vi "Autonomous Independent.vi"() -> ()   [LabVIEW 2013]
doc: "This VI is called when autonomous begins, and will automatically be terminated when autonomous ends. You can carry out timed or sensor driven robot movement independently without needing to return to the caller."
uses:
  Systems/DriveMotors/DriveMotors.lvclass
  Systems/GrabberWheels/GrabberWheels.lvclass
  Systems/GrabberArms/GrabberArms.lvclass
  Commands/Command/Command.lvclass
  Systems/Catapult/Catapult.lvclass
  Commands/CT-De-energize-Command/CT-De-energize-Cmd.lvclass
  Systems/Blocker/Blocker.lvclass
  Commands/DM-DriveForwardDistance/DM-DriveForwardDistance.lvclass
  Robot Global Data.vi
  Commands/GA-Extend-Command/GA-Extend-Cmd.lvclass
  Commands/BL-Extend-Command/BL-Extend-Cmd.lvclass
  Commands/GW-SpitOut-Command/GW-SpitOut-Cmd.lvclass
  Commands/GW-Stop-Command/GW-Stop-Cmd.lvclass
panel:
  in  "Time to Settle(ms)":u32=500
  in  "Time to Spit Out":u32
  out "AutoMode: Drive Forward and Shoot":bool
  in  "Use PID":bool
  out "Right Power":dbl
  in  "Trim":dbl(knob) step=0.001 scale=0.0..0.25
  in  "Test Wait":u32=25
  in  "DrivePower":dbl=0.6 format="%#_13g"
  # "Be sure to right-click and choose Data Operations>>Make Current Value default if you want to save the array values with the VI"
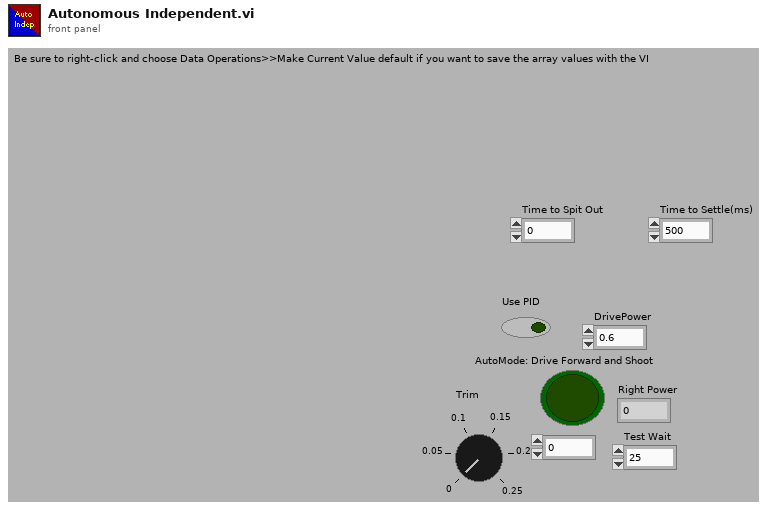
[diagram p1: front panel]
types:
  T1 = typedef "Semaphore RefNum" = refnum<k1>
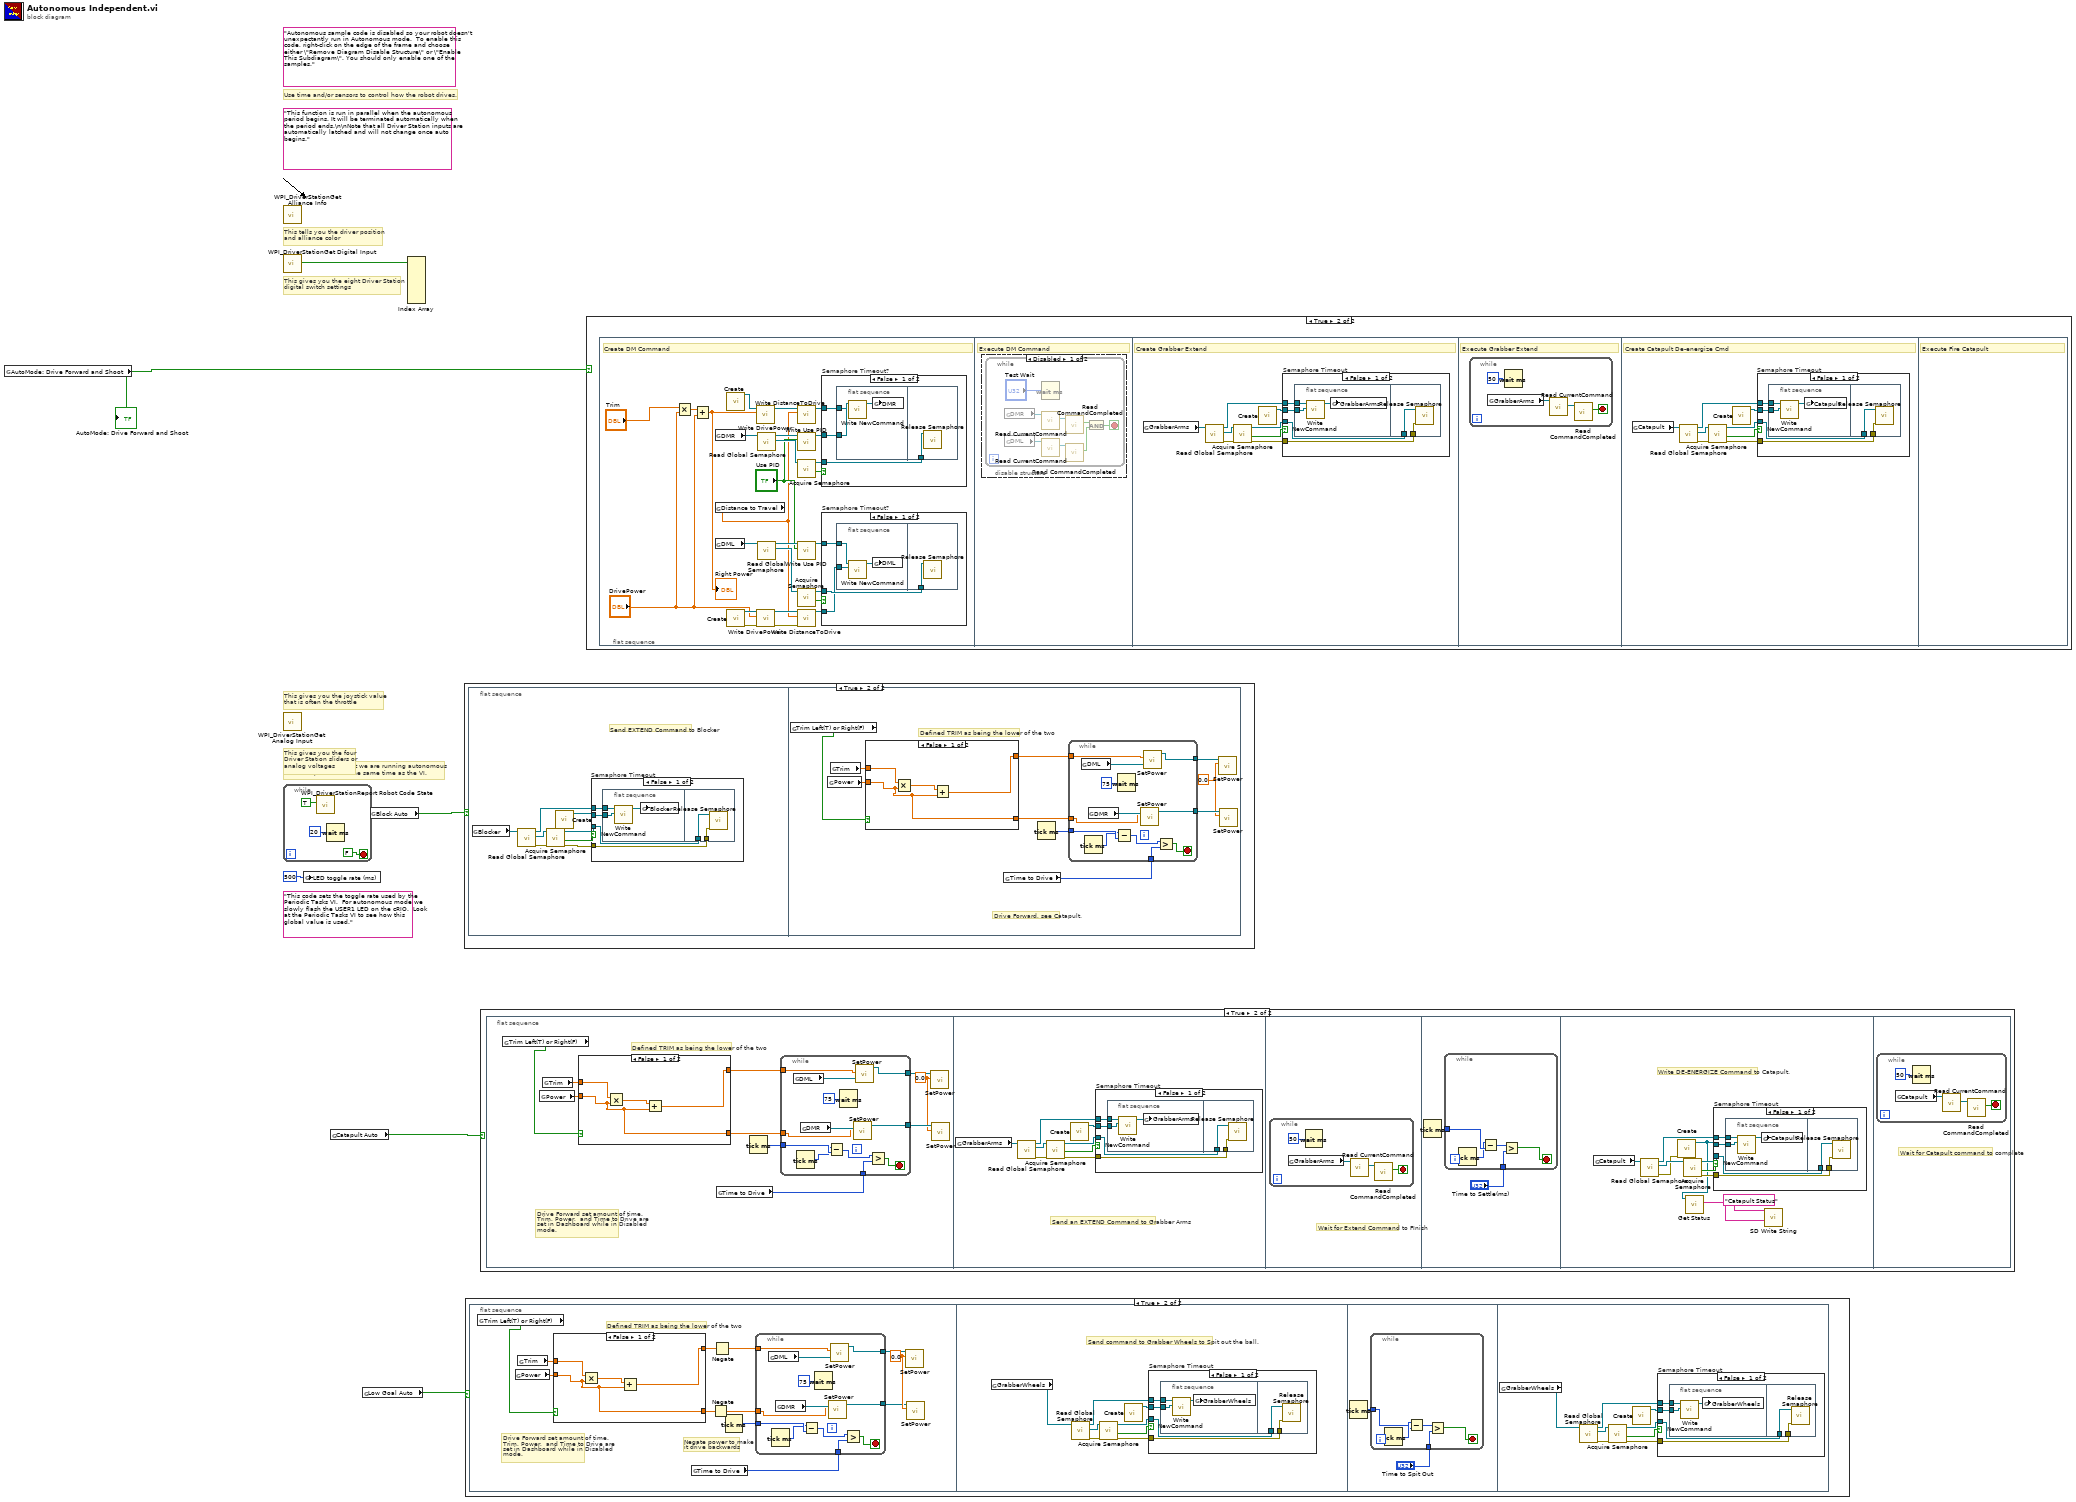
[diagram p0: block diagram]
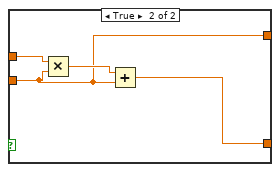
[diagram p3: hidden frame]
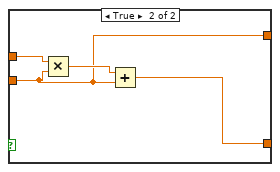
[diagram p7: hidden frame]
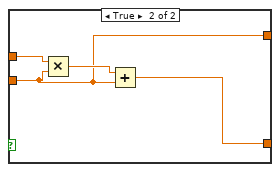
[diagram p12: hidden frame]
diagram:
  (unwired) "This code sets the toggle rate used by the Periodic Tasks VI.  For autonomous mode we slowly flash the USER1 LED on the cRIO.  Look at the Periodic Tasks VI to see how this global value is used."
  (unwired) "Autonomous sample code is disabled so your robot doesn't unexpectantly run in Autonomous mode.  To enable this code, right-click on the edge of the frame and choose either \"Remove Diagram Disable Structure\" or \"Enable This Subdiagram\". You should only enable one of the samples."
  (unwired) "This function is run in parallel when the autonomous period begins. It will be terminated automatically when the period ends.\n\nNote that all Driver Station inputs are automatically latched and will not change once auto begins."
  # "Every 20ms, report that we are running autonomous\ncode. Loop will abort the same time as the VI."
  # "This gives you the joystick value\nthat is often the throttle"
  # "Use time and/or sensors to control how the robot drives."
  # "This tells you the driver position\nand alliance color"
  # "This gives you the eight Driver Station\ndigital switch settings"
  # "This gives you the four\nDriver Station sliders or\nanalog voltages"
  n1 = global read "Robot Global Data.vi" "AutoMode: Drive Forward and Shoot"() -> (w4:bool)
  "AutoMode: Drive Forward and Shoot" <- w4
  n2 = call <vilib>:"WPI_DriverStationGet Alliance Info.vi"() -> ()  [unwired: 12 out]
  n3 = call <vilib>:"WPI_DriverStationGet Digital Input.vi"() -> ("Driver Station Digital Input (1-8)"=w6:bool[])  [unwired: 11 out]
  n4 = call <vilib>:"WPI_DriverStationGet Analog Input.vi"() -> ()  [unwired: 12 out]
  n5 = while {
    stop <- FALSE stop-if-true
    n6 = call <vilib>:"WPI_DriverStationReport Robot Code State.vi"("Autonomous"=TRUE) -> ()  [unwired: 10 in, 1 out]
    n7 = Wait (ms)(milliseconds to wait=u32 20) -> ()  [unwired: 1 out]
  }
  n8 = global write "Robot Global Data.vi" "LED toggle rate (ms)"(u32 500 ("LED ms toggle rate")) -> ()
  n9 = global read "Robot Global Data.vi" "Catapult Auto"() -> (w2:bool)
  n10 = global read "Robot Global Data.vi" "Low Goal Auto"() -> (w1:bool)
  n11 = global read "Robot Global Data.vi" "Block Auto"() -> (w3:bool)
  n12 = Index Array(array=w6) -> ()  [unwired: 8 in, 8 out]
  n13 = case shown="True" w3 {
    frame False {
    }
    frame True {
      n14 = flat-sequence {
        frame #0 {
          # "Send EXTEND Command to Blocker"
          n15 = global read "Robot Global Data.vi" "Blocker"() -> (w17:refnum<class "Blocker.lvclass">)
          n16 = call-dynamic "Read Global Semaphore.vi"("System in"=w17) -> ("error out"=w14:errorcluster, "semaphore"=w15:T1, "System out"=w16:refnum<class "Blocker.lvclass">)  [unwired: 8 in]
          n17 = call <vilib>:"Acquire Semaphore.vi"("error in (no error)"=w14, "semaphore"=w15) -> ("error out"=w12:errorcluster, "timed out"=w11:bool, "semaphore out"=w13:T1)  [unwired: 3 in]
          n18 = call "Create.vi"() -> ("BL-Extend-Cmd out"=w10:refnum<class "BL-Extend-Cmd.lvclass">)  [unwired: 10 in, 1 out]
          n19 = case "Semaphore Timeout" shown="False" w11 {
            tunnel: w16 -> [w21 _]
            tunnel: w13 -> [w20 _]
            tunnel: w12 -> [w19 _]
            tunnel: w10 -> [w18 _]
            frame False {
              n20 = flat-sequence {
                tunnel: w21 -> [w23]
                tunnel: w18 -> [w22]
                tunnel: w20 -> [w26]
                tunnel: w19 -> [w25]
                frame #0 {
                  n21 = call-dynamic "Write NewCommand.vi"("Command.lvclass"=w22, "System in"=w23) -> ("System out"=w24:refnum<class "Blocker.lvclass">)  [unwired: 8 in, 1 out]
                  n22 = global write "Robot Global Data.vi" "Blocker"(w24) -> ()
                }
                frame #1 {
                  n23 = call <vilib>:"Release Semaphore.vi"("error in (no error)"=w25, "semaphore"=w26) -> ()  [unwired: 4 in, 2 out]
                }
              }
            }
            frame True {
            }
          }
        }
        frame #1 {
          w33 = 0.0 ("MotorPower Terminal")
          # "Drive Forward, see Catapult."
          # "Defined TRIM as being the lower of the two"
          n24 = global read "Robot Global Data.vi" "Trim Left(T) or Right(F)"() -> (w32:bool)
          n25 = global read "Robot Global Data.vi" "Power"() -> (w30:dbl)
          n26 = global read "Robot Global Data.vi" "Trim"() -> (w31:dbl)
          n27 = case shown="False" w32 {
            tunnel: w31 -> [w39 w44]
            tunnel: w30 -> [w37 w41]
            tunnel: [w37 w42] -> w29
            tunnel: [w38 w41] -> w28
            frame False {
              n28 = Multiply(x=w39, y=w37) -> (x*y=w40:dbl)
              n29 = Add(x=w40, y=w37) -> (x+y=w38:dbl)
            }
            frame True {
              n30 = Multiply(x=w44, y=w41) -> (x*y=w43:dbl)
              n31 = Add(x=w43, y=w41) -> (x+y=w42:dbl)
            }
          }
          n32 = global read "Robot Global Data.vi" "Time to Drive"() -> (w27:u32)
          n33 = Tick Count (ms)() -> (millisecond timer value=w36:u32)
          n34 = while {
            tunnel: w36 -> [w54]
            tunnel: [w51] -> w35
            tunnel: [w50] -> w34
            tunnel: w29 -> [w48]
            tunnel: w28 -> [w47]
            tunnel: w27 -> [w46]
            stop <- w49 stop-if-true
            n35 = global read "Robot Global Data.vi" "DML"() -> (w55:refnum<class "DriveMotors.lvclass">)
            n36 = Tick Count (ms)() -> (millisecond timer value=w53:u32)
            n37 = global read "Robot Global Data.vi" "DMR"() -> (w56:refnum<class "DriveMotors.lvclass">)
            n38 = Subtract(x=w53, y=w54) -> (x-y=w52:u32)
            n39 = Wait (ms)(milliseconds to wait=u32 75) -> ()  [unwired: 1 out]
            n40 = call-dynamic "SetPower.vi"("MotorPower Terminal"=w48, "DriveMotors in"=w56) -> ("DriveMotors out"=w51:refnum<class "DriveMotors.lvclass">)  [unwired: 8 in, 1 out]
            n41 = call-dynamic "SetPower.vi"("MotorPower Terminal"=w47, "DriveMotors in"=w55) -> ("DriveMotors out"=w50:refnum<class "DriveMotors.lvclass">)  [unwired: 8 in, 1 out]
            n42 = Greater?(x=w52, y=w46) -> (0:w49:bool)
          }
          n43 = call-dynamic "SetPower.vi"("MotorPower Terminal"=w33, "DriveMotors in"=w34) -> ()  [unwired: 8 in, 2 out]
          n44 = call-dynamic "SetPower.vi"("MotorPower Terminal"=w33, "DriveMotors in"=w35) -> ()  [unwired: 8 in, 2 out]
        }
      }
    }
  }
  n45 = case shown="True" w1 {
    frame False {
    }
    frame True {
      n46 = flat-sequence {
        frame #0 {
          w62 = 0.0 ("MotorPower Terminal")
          # "Negate power to make \nit drive backwards"
          # "Drive Forward set amount of time.\nTrim, Power,  and Time to Drive are \nset in Dashboard while in Disabled \nmode."
          # "Defined TRIM as being the lower of the two"
          n47 = global read "Robot Global Data.vi" "Trim Left(T) or Right(F)"() -> (w63:bool)
          n48 = global read "Robot Global Data.vi" "Power"() -> (w65:dbl)
          n49 = global read "Robot Global Data.vi" "Trim"() -> (w64:dbl)
          n50 = case shown="False" w63 {
            tunnel: w64 -> [w71 w76]
            tunnel: w65 -> [w69 w73]
            tunnel: [w69 w74] -> w66
            tunnel: [w70 w73] -> w67
            frame False {
              n51 = Multiply(x=w71, y=w69) -> (x*y=w72:dbl)
              n52 = Add(x=w72, y=w69) -> (x+y=w70:dbl)
            }
            frame True {
              n53 = Multiply(x=w76, y=w73) -> (x*y=w75:dbl)
              n54 = Add(x=w75, y=w73) -> (x+y=w74:dbl)
            }
          }
          n55 = global read "Robot Global Data.vi" "Time to Drive"() -> (w68:u32)
          n56 = Negate(x=w66) -> (-x=w57:dbl)
          n57 = Negate(x=w67) -> (-x=w58:dbl)
          n58 = Tick Count (ms)() -> (millisecond timer value=w59:u32)
          n59 = while {
            tunnel: w59 -> [w86]
            tunnel: [w83] -> w60
            tunnel: [w82] -> w61
            tunnel: w57 -> [w80]
            tunnel: w58 -> [w79]
            tunnel: w68 -> [w78]
            stop <- w81 stop-if-true
            n60 = global read "Robot Global Data.vi" "DML"() -> (w87:refnum<class "DriveMotors.lvclass">)
            n61 = Tick Count (ms)() -> (millisecond timer value=w85:u32)
            n62 = global read "Robot Global Data.vi" "DMR"() -> (w88:refnum<class "DriveMotors.lvclass">)
            n63 = Subtract(x=w85, y=w86) -> (x-y=w84:u32)
            n64 = Wait (ms)(milliseconds to wait=u32 75) -> ()  [unwired: 1 out]
            n65 = call-dynamic "SetPower.vi"("MotorPower Terminal"=w80, "DriveMotors in"=w88) -> ("DriveMotors out"=w83:refnum<class "DriveMotors.lvclass">)  [unwired: 8 in, 1 out]
            n66 = call-dynamic "SetPower.vi"("MotorPower Terminal"=w79, "DriveMotors in"=w87) -> ("DriveMotors out"=w82:refnum<class "DriveMotors.lvclass">)  [unwired: 8 in, 1 out]
            n67 = Greater?(x=w84, y=w78) -> (0:w81:bool)
          }
          n68 = call-dynamic "SetPower.vi"("MotorPower Terminal"=w62, "DriveMotors in"=w61) -> ()  [unwired: 8 in, 2 out]
          n69 = call-dynamic "SetPower.vi"("MotorPower Terminal"=w62, "DriveMotors in"=w60) -> ()  [unwired: 8 in, 2 out]
        }
        frame #1 {
          # "Send command to Grabber Wheels to Spit out the ball."
          n70 = global read "Robot Global Data.vi" "GrabberWheels"() -> (w89:refnum<class "GrabberWheels.lvclass">)
          n71 = call-dynamic "Read Global Semaphore.vi"("System in"=w89) -> ("error out"=w92:errorcluster, "semaphore"=w91:T1, "System out"=w90:refnum<class "GrabberWheels.lvclass">)  [unwired: 8 in]
          n72 = call <vilib>:"Acquire Semaphore.vi"("error in (no error)"=w92, "semaphore"=w91) -> ("error out"=w95:errorcluster, "timed out"=w93:bool, "semaphore out"=w94:T1)  [unwired: 3 in]
          n73 = call "Create.vi"() -> ("GW-SpitOut-Cmd out"=w96:refnum<class "GW-SpitOut-Cmd.lvclass">)  [unwired: 10 in, 1 out]
          n74 = case "Semaphore Timeout" shown="False" w93 {
            tunnel: w90 -> [w100 _]
            tunnel: w94 -> [w99 _]
            tunnel: w95 -> [w98 _]
            tunnel: w96 -> [w97 _]
            frame False {
              n75 = flat-sequence {
                tunnel: w100 -> [w102]
                tunnel: w97 -> [w101]
                tunnel: w99 -> [w105]
                tunnel: w98 -> [w104]
                frame #0 {
                  n76 = call-dynamic "Write NewCommand.vi"("Command.lvclass"=w101, "System in"=w102) -> ("System out"=w103:refnum<class "GrabberWheels.lvclass">)  [unwired: 8 in, 1 out]
                  n77 = global write "Robot Global Data.vi" "GrabberWheels"(w103) -> ()
                }
                frame #1 {
                  n78 = call <vilib>:"Release Semaphore.vi"("error in (no error)"=w104, "semaphore"=w105) -> ()  [unwired: 4 in, 2 out]
                }
              }
            }
            frame True {
            }
          }
        }
        frame #2 {
          n79 = Tick Count (ms)() -> (millisecond timer value=w107:u32)
          n80 = while {
            tunnel: w107 -> [w108]
            tunnel: "Time to Spit Out" -> [w110]
            stop <- w111 stop-if-true
            n81 = Tick Count (ms)() -> (millisecond timer value=w109:u32)
            n82 = Subtract(x=w109, y=w108) -> (x-y=w112:u32)
            n83 = Greater?(x=w112, y=w110) -> (0:w111:bool)
          }
        }
        frame #3 {
          n84 = global read "Robot Global Data.vi" "GrabberWheels"() -> (w113:refnum<class "GrabberWheels.lvclass">)
          n85 = call-dynamic "Read Global Semaphore.vi"("System in"=w113) -> ("error out"=w116:errorcluster, "semaphore"=w115:T1, "System out"=w114:refnum<class "GrabberWheels.lvclass">)  [unwired: 8 in]
          n86 = call <vilib>:"Acquire Semaphore.vi"("error in (no error)"=w116, "semaphore"=w115) -> ("error out"=w119:errorcluster, "timed out"=w117:bool, "semaphore out"=w118:T1)  [unwired: 3 in]
          n87 = call "Create.vi"() -> ("GW-Stop-Cmd out"=w120:refnum<class "GW-Stop-Cmd.lvclass">)  [unwired: 10 in, 1 out]
          n88 = case "Semaphore Timeout" shown="False" w117 {
            tunnel: w114 -> [w124 _]
            tunnel: w118 -> [w123 _]
            tunnel: w119 -> [w122 _]
            tunnel: w120 -> [w121 _]
            frame False {
              n89 = flat-sequence {
                tunnel: w124 -> [w126]
                tunnel: w121 -> [w125]
                tunnel: w123 -> [w129]
                tunnel: w122 -> [w128]
                frame #0 {
                  n90 = call-dynamic "Write NewCommand.vi"("Command.lvclass"=w125, "System in"=w126) -> ("System out"=w127:refnum<class "GrabberWheels.lvclass">)  [unwired: 8 in, 1 out]
                  n91 = global write "Robot Global Data.vi" "GrabberWheels"(w127) -> ()
                }
                frame #1 {
                  n92 = call <vilib>:"Release Semaphore.vi"("error in (no error)"=w128, "semaphore"=w129) -> ()  [unwired: 4 in, 2 out]
                }
              }
            }
            frame True {
            }
          }
        }
      }
    }
  }
  n93 = case shown="True" w2 {
    frame False {
    }
    frame True {
      n94 = flat-sequence {
        frame #0 {
          w136 = 0.0 ("MotorPower Terminal")
          # "Drive Forward set amount of time.\nTrim, Power,  and Time to Drive are \nset in Dashboard while in Disabled \nmode."
          # "Defined TRIM as being the lower of the two"
          n95 = global read "Robot Global Data.vi" "Trim Left(T) or Right(F)"() -> (w135:bool)
          n96 = global read "Robot Global Data.vi" "Power"() -> (w133:dbl)
          n97 = global read "Robot Global Data.vi" "Trim"() -> (w134:dbl)
          n98 = case shown="False" w135 {
            tunnel: w134 -> [w142 w147]
            tunnel: w133 -> [w140 w144]
            tunnel: [w140 w145] -> w132
            tunnel: [w141 w144] -> w131
            frame False {
              n99 = Multiply(x=w142, y=w140) -> (x*y=w143:dbl)
              n100 = Add(x=w143, y=w140) -> (x+y=w141:dbl)
            }
            frame True {
              n101 = Multiply(x=w147, y=w144) -> (x*y=w146:dbl)
              n102 = Add(x=w146, y=w144) -> (x+y=w145:dbl)
            }
          }
          n103 = global read "Robot Global Data.vi" "Time to Drive"() -> (w130:u32)
          n104 = Tick Count (ms)() -> (millisecond timer value=w139:u32)
          n105 = while {
            tunnel: w139 -> [w157]
            tunnel: [w154] -> w138
            tunnel: [w153] -> w137
            tunnel: w132 -> [w151]
            tunnel: w131 -> [w150]
            tunnel: w130 -> [w149]
            stop <- w152 stop-if-true
            n106 = global read "Robot Global Data.vi" "DML"() -> (w158:refnum<class "DriveMotors.lvclass">)
            n107 = Tick Count (ms)() -> (millisecond timer value=w156:u32)
            n108 = global read "Robot Global Data.vi" "DMR"() -> (w159:refnum<class "DriveMotors.lvclass">)
            n109 = Subtract(x=w156, y=w157) -> (x-y=w155:u32)
            n110 = Wait (ms)(milliseconds to wait=u32 75) -> ()  [unwired: 1 out]
            n111 = call-dynamic "SetPower.vi"("MotorPower Terminal"=w151, "DriveMotors in"=w159) -> ("DriveMotors out"=w154:refnum<class "DriveMotors.lvclass">)  [unwired: 8 in, 1 out]
            n112 = call-dynamic "SetPower.vi"("MotorPower Terminal"=w150, "DriveMotors in"=w158) -> ("DriveMotors out"=w153:refnum<class "DriveMotors.lvclass">)  [unwired: 8 in, 1 out]
            n113 = Greater?(x=w155, y=w149) -> (0:w152:bool)
          }
          n114 = call-dynamic "SetPower.vi"("MotorPower Terminal"=w136, "DriveMotors in"=w137) -> ()  [unwired: 8 in, 2 out]
          n115 = call-dynamic "SetPower.vi"("MotorPower Terminal"=w136, "DriveMotors in"=w138) -> ()  [unwired: 8 in, 2 out]
        }
        frame #1 {
          # "Send an EXTEND Command to Grabber Arms"
          n116 = global read "Robot Global Data.vi" "GrabberArms"() -> (w167:refnum<class "GrabberArms.lvclass">)
          n117 = call-dynamic "Read Global Semaphore.vi"("System in"=w167) -> ("error out"=w164:errorcluster, "semaphore"=w165:T1, "System out"=w166:refnum<class "GrabberArms.lvclass">)  [unwired: 8 in]
          n118 = call <vilib>:"Acquire Semaphore.vi"("error in (no error)"=w164, "semaphore"=w165) -> ("error out"=w161:errorcluster, "timed out"=w163:bool, "semaphore out"=w162:T1)  [unwired: 3 in]
          n119 = call "Create.vi"() -> ("GA-Extend-Cmd out"=w160:refnum<class "GA-Extend-Cmd.lvclass">)  [unwired: 10 in, 1 out]
          n120 = case "Semaphore Timeout" shown="False" w163 {
            tunnel: w166 -> [w171 _]
            tunnel: w162 -> [w170 _]
            tunnel: w161 -> [w169 _]
            tunnel: w160 -> [w168 _]
            frame False {
              n121 = flat-sequence {
                tunnel: w171 -> [w173]
                tunnel: w168 -> [w172]
                tunnel: w170 -> [w176]
                tunnel: w169 -> [w175]
                frame #0 {
                  n122 = call-dynamic "Write NewCommand.vi"("Command.lvclass"=w172, "System in"=w173) -> ("System out"=w174:refnum<class "GrabberArms.lvclass">)  [unwired: 8 in, 1 out]
                  n123 = global write "Robot Global Data.vi" "GrabberArms"(w174) -> ()
                }
                frame #1 {
                  n124 = call <vilib>:"Release Semaphore.vi"("error in (no error)"=w175, "semaphore"=w176) -> ()  [unwired: 4 in, 2 out]
                }
              }
            }
            frame True {
            }
          }
        }
        frame #2 {
          # "Wait for Extend Command to FInish"
          n125 = while {
            stop <- w177 stop-if-true
            n126 = global read "Robot Global Data.vi" "GrabberArms"() -> (w178:refnum<class "GrabberArms.lvclass">)
            n127 = Wait (ms)(milliseconds to wait=u32 50) -> ()  [unwired: 1 out]
            n128 = call-dynamic "Read CurrentCommand.vi"("System in"=w178) -> ("Command.lvclass"=w179:refnum<class "Command.lvclass">)  [unwired: 8 in, 2 out]
            n129 = call-dynamic "Read CommandCompleted.vi"("Command in"=w179) -> ("CommandCompleted"=w177:bool)  [unwired: 8 in, 2 out]
          }
        }
        frame #3 {
          n130 = Tick Count (ms)() -> (millisecond timer value=w182:u32)
          n131 = while {
            tunnel: w182 -> [w184]
            tunnel: "Time to Settle(ms)" -> [w185]
            stop <- w186 stop-if-true
            n132 = Tick Count (ms)() -> (millisecond timer value=w183:u32)
            n133 = Subtract(x=w183, y=w184) -> (x-y=w187:u32)
            n134 = Greater?(x=w187, y=w185) -> (0:w186:bool)
          }
        }
        frame #4 {
          # "Write DE-ENERGIZE Command to Catapult."
          n135 = global read "Robot Global Data.vi" "Catapult"() -> (w198:refnum<class "Catapult.lvclass">)
          n136 = call-dynamic "Read Global Semaphore.vi"("System in"=w198) -> ("error out"=w189:errorcluster, "semaphore"=w196:T1, "System out"=w197:refnum<class "Catapult.lvclass">)  [unwired: 8 in]
          n137 = call "Create.vi"("error in (no error)"=w189) -> ("error out"=w188:errorcluster, "CT-De-energize-Cmd.lvclass"=w192:refnum<class "CT-De-energize-Cmd.lvclass">)  [unwired: 9 in]
          n138 = call <vilib>:"Acquire Semaphore.vi"("error in (no error)"=w188, "semaphore"=w196) -> ("error out"=w194:errorcluster, "timed out"=w193:bool, "semaphore out"=w195:T1)  [unwired: 3 in]
          n139 = call-dynamic "Get Status.vi"("Command in"=w192) -> ("Status"=w191:string)  [unwired: 8 in, 2 out]
          n140 = case "Semaphore Timeout" shown="False" w193 {
            tunnel: w197 -> [w202 _]
            tunnel: w195 -> [w201 _]
            tunnel: w194 -> [w200 _]
            tunnel: w192 -> [w199 _]
            frame False {
              n141 = flat-sequence {
                tunnel: w202 -> [w204]
                tunnel: w199 -> [w203]
                tunnel: w201 -> [w207]
                tunnel: w200 -> [w206]
                frame #0 {
                  n142 = call-dynamic "Write NewCommand.vi"("Command.lvclass"=w203, "System in"=w204) -> ("System out"=w205:refnum<class "Catapult.lvclass">)  [unwired: 8 in, 1 out]
                  n143 = global write "Robot Global Data.vi" "Catapult"(w205) -> ()
                }
                frame #1 {
                  n144 = call <vilib>:"Release Semaphore.vi"("error in (no error)"=w206, "semaphore"=w207) -> ()  [unwired: 4 in, 2 out]
                }
              }
            }
            frame True {
            }
          }
          n145 = call <vilib>:"SD Write String.vi"("String"=w191, "Name"="Catapult Status") -> ()  [unwired: 8 in, 2 out]
        }
        frame #5 {
          # "Wait for Catapult command to complete"
          n146 = while {
            stop <- w208 stop-if-true
            n147 = global read "Robot Global Data.vi" "Catapult"() -> (w209:refnum<class "Catapult.lvclass">)
            n148 = Wait (ms)(milliseconds to wait=u32 50) -> ()  [unwired: 1 out]
            n149 = call-dynamic "Read CurrentCommand.vi"("System in"=w209) -> ("Command.lvclass"=w210:refnum<class "Command.lvclass">)  [unwired: 8 in, 2 out]
            n150 = call-dynamic "Read CommandCompleted.vi"("Command in"=w210) -> ("CommandCompleted"=w208:bool)  [unwired: 8 in, 2 out]
          }
        }
      }
    }
  }
  n151 = case shown="True" w4 {
    frame False {
    }
    frame True {
      n152 = flat-sequence {
        frame #0 {
          # "Create DM Command"
          n153 = Multiply(x="Trim", y="DrivePower") -> (x*y=w219:dbl)
          n154 = Add(x=w219, y="DrivePower") -> (x+y=w218:dbl)
          "Right Power" <- w218
          n155 = global read "Robot Global Data.vi" "DMR"() -> (w235:refnum<class "DriveMotors.lvclass">)
          n156 = global read "Robot Global Data.vi" "Distance to Travel"() -> (w212:dbl)
          n157 = global read "Robot Global Data.vi" "DML"() -> (w229:refnum<class "DriveMotors.lvclass">)
          n158 = call "Create.vi"() -> ("DM-DriveForwardDistance.lvclass"=w224:refnum<class "DM-DriveForwardDistance.lvclass">)  [unwired: 10 in, 1 out]
          n159 = call "Create.vi"() -> ("error out"=w231:errorcluster, "DM-DriveForwardDistance.lvclass"=w237:refnum<class "DM-DriveForwardDistance.lvclass">)  [unwired: 10 in]
          n160 = call-dynamic "Write DrivePower.vi"("DrivePower"=w218, "DM-DriveForwardDistance in"=w224) -> ("DM-DriveForwardDistance out"=w223:refnum<class "DM-DriveForwardDistance.lvclass">)  [unwired: 8 in, 1 out]
          n161 = call-dynamic "Write DrivePower.vi"("error in (no error)"=w231, "DrivePower"="DrivePower", "DM-DriveForwardDistance in"=w237) -> ("error out"=w230:errorcluster, "DM-DriveForwardDistance out"=w236:refnum<class "DM-DriveForwardDistance.lvclass">)  [unwired: 7 in]
          n162 = call-dynamic "Read Global Semaphore.vi"("System in"=w235) -> ("semaphore"=w234:T1, "System out"=w217:refnum<class "DriveMotors.lvclass">)  [unwired: 8 in, 1 out]
          n163 = call-dynamic "Read Global Semaphore.vi"("System in"=w229) -> ("semaphore"=w228:T1, "System out"=w215:refnum<class "DriveMotors.lvclass">)  [unwired: 8 in, 1 out]
          n164 = call-dynamic "Write DistanceToDrive.vi"("DistanceToDrive"=w212, "DM-DriveForwardDistance in"=w223) -> ("DM-DriveForwardDistance out"=w222:refnum<class "DM-DriveForwardDistance.lvclass">)  [unwired: 8 in, 1 out]
          n165 = call-dynamic "Write Use PID.vi"("Use PID"="Use PID", "DriveMotors in"=w217) -> ("DriveMotors out"=w216:refnum<class "DriveMotors.lvclass">)  [unwired: 8 in, 1 out]
          n166 = call <vilib>:"Acquire Semaphore.vi"("semaphore"=w234) -> ("timed out"=w233:bool, "semaphore out"=w232:T1)  [unwired: 4 in, 1 out]
          n167 = call-dynamic "Write Use PID.vi"("Use PID"="Use PID", "DriveMotors in"=w215) -> ("DriveMotors out"=w214:refnum<class "DriveMotors.lvclass">)  [unwired: 8 in, 1 out]
          n168 = call <vilib>:"Acquire Semaphore.vi"("semaphore"=w228) -> ("timed out"=w226:bool, "semaphore out"=w227:T1)  [unwired: 4 in, 1 out]
          n169 = call-dynamic "Write DistanceToDrive.vi"("error in (no error)"=w230, "DistanceToDrive"=w212, "DM-DriveForwardDistance in"=w236) -> ("DM-DriveForwardDistance out"=w225:refnum<class "DM-DriveForwardDistance.lvclass">)  [unwired: 7 in, 1 out]
          n170 = case "Semaphore Timeout?" shown="False" w233 {
            tunnel: w216 -> [w247 _]
            tunnel: w222 -> [w246 _]
            tunnel: w232 -> [w245 _]
            frame False {
              n171 = flat-sequence {
                tunnel: w247 -> [w250]
                tunnel: w246 -> [w249]
                tunnel: w245 -> [w251]
                frame #0 {
                  n172 = call-dynamic "Write NewCommand.vi"("Command.lvclass"=w249, "System in"=w250) -> ("System out"=w248:refnum<class "DriveMotors.lvclass">)  [unwired: 8 in, 1 out]
                  n173 = global write "Robot Global Data.vi" "DMR"(w248) -> ()
                }
                frame #1 {
                  n174 = call <vilib>:"Release Semaphore.vi"("semaphore"=w251) -> ()  [unwired: 5 in, 2 out]
                }
              }
            }
            frame True {
            }
          }
          n175 = case "Semaphore Timeout?" shown="False" w226 {
            tunnel: w214 -> [w240 _]
            tunnel: w227 -> [w239 _]
            tunnel: w225 -> [w238 _]
            frame False {
              n176 = flat-sequence {
                tunnel: w240 -> [w243]
                tunnel: w238 -> [w242]
                tunnel: w239 -> [w244]
                frame #0 {
                  n177 = call-dynamic "Write NewCommand.vi"("Command.lvclass"=w242, "System in"=w243) -> ("System out"=w241:refnum<class "DriveMotors.lvclass">)  [unwired: 8 in, 1 out]
                  n178 = global write "Robot Global Data.vi" "DML"(w241) -> ()
                }
                frame #1 {
                  n179 = call <vilib>:"Release Semaphore.vi"("semaphore"=w244) -> ()  [unwired: 5 in, 2 out]
                }
              }
            }
            frame True {
            }
          }
        }
        frame #1 {
          # "Execute DM Command"
          n180 = disable-structure shown="Disabled" {
            frame Disabled {
              n181 = while {
                stop <- w253 stop-if-true
                n182 = global read "Robot Global Data.vi" "DMR"() -> (w256:refnum<class "DriveMotors.lvclass">)
                n183 = global read "Robot Global Data.vi" "DML"() -> (w255:refnum<class "DriveMotors.lvclass">)
                n184 = Wait (ms)(milliseconds to wait="Test Wait") -> ()  [unwired: 1 out]
                n185 = call-dynamic "Read CurrentCommand.vi"("System in"=w256) -> ("Command.lvclass"=w258:refnum<class "Command.lvclass">)  [unwired: 8 in, 2 out]
                n186 = call-dynamic "Read CurrentCommand.vi"("System in"=w255) -> ("Command.lvclass"=w254:refnum<class "Command.lvclass">)  [unwired: 8 in, 2 out]
                n187 = call-dynamic "Read CommandCompleted.vi"("Command in"=w258) -> ("CommandCompleted"=w257:bool)  [unwired: 8 in, 2 out]
                n188 = call-dynamic "Read CommandCompleted.vi"("Command in"=w254) -> ("CommandCompleted"=w252:bool)  [unwired: 8 in, 2 out]
                n189 = And(x=w257, y=w252) -> (x .and. y?=w253:bool)
              }
            }
            frame Enabled {
            }
          }
        }
        frame #2 {
          # "Create Grabber Extend"
          n190 = global read "Robot Global Data.vi" "GrabberArms"() -> (w267:refnum<class "GrabberArms.lvclass">)
          n191 = call-dynamic "Read Global Semaphore.vi"("System in"=w267) -> ("error out"=w264:errorcluster, "semaphore"=w265:T1, "System out"=w266:refnum<class "GrabberArms.lvclass">)  [unwired: 8 in]
          n192 = call <vilib>:"Acquire Semaphore.vi"("error in (no error)"=w264, "semaphore"=w265) -> ("error out"=w261:errorcluster, "timed out"=w263:bool, "semaphore out"=w262:T1)  [unwired: 3 in]
          n193 = call "Create.vi"() -> ("GA-Extend-Cmd out"=w260:refnum<class "GA-Extend-Cmd.lvclass">)  [unwired: 10 in, 1 out]
          n194 = case "Semaphore Timeout" shown="False" w263 {
            tunnel: w266 -> [w271 _]
            tunnel: w262 -> [w270 _]
            tunnel: w261 -> [w269 _]
            tunnel: w260 -> [w268 _]
            frame False {
              n195 = flat-sequence {
                tunnel: w271 -> [w273]
                tunnel: w268 -> [w272]
                tunnel: w270 -> [w276]
                tunnel: w269 -> [w275]
                frame #0 {
                  n196 = call-dynamic "Write NewCommand.vi"("Command.lvclass"=w272, "System in"=w273) -> ("System out"=w274:refnum<class "GrabberArms.lvclass">)  [unwired: 8 in, 1 out]
                  n197 = global write "Robot Global Data.vi" "GrabberArms"(w274) -> ()
                }
                frame #1 {
                  n198 = call <vilib>:"Release Semaphore.vi"("error in (no error)"=w275, "semaphore"=w276) -> ()  [unwired: 4 in, 2 out]
                }
              }
            }
            frame True {
            }
          }
        }
        frame #3 {
          # "Execute Grabber Extend"
          n199 = while {
            stop <- w277 stop-if-true
            n200 = global read "Robot Global Data.vi" "GrabberArms"() -> (w278:refnum<class "GrabberArms.lvclass">)
            n201 = Wait (ms)(milliseconds to wait=u32 50) -> ()  [unwired: 1 out]
            n202 = call-dynamic "Read CurrentCommand.vi"("System in"=w278) -> ("Command.lvclass"=w279:refnum<class "Command.lvclass">)  [unwired: 8 in, 2 out]
            n203 = call-dynamic "Read CommandCompleted.vi"("Command in"=w279) -> ("CommandCompleted"=w277:bool)  [unwired: 8 in, 2 out]
          }
        }
        frame #4 {
          # "Create Catapult De-energize Cmd"
          n204 = global read "Robot Global Data.vi" "Catapult"() -> (w288:refnum<class "Catapult.lvclass">)
          n205 = call-dynamic "Read Global Semaphore.vi"("System in"=w288) -> ("error out"=w285:errorcluster, "semaphore"=w286:T1, "System out"=w287:refnum<class "Catapult.lvclass">)  [unwired: 8 in]
          n206 = call <vilib>:"Acquire Semaphore.vi"("error in (no error)"=w285, "semaphore"=w286) -> ("error out"=w283:errorcluster, "timed out"=w282:bool, "semaphore out"=w284:T1)  [unwired: 3 in]
          n207 = call "Create.vi"() -> ("CT-De-energize-Cmd.lvclass"=w281:refnum<class "CT-De-energize-Cmd.lvclass">)  [unwired: 10 in, 1 out]
          n208 = case "Semaphore Timeout" shown="False" w282 {
            tunnel: w287 -> [w292 _]
            tunnel: w284 -> [w291 _]
            tunnel: w283 -> [w290 _]
            tunnel: w281 -> [w289 _]
            frame False {
              n209 = flat-sequence {
                tunnel: w292 -> [w294]
                tunnel: w289 -> [w293]
                tunnel: w291 -> [w297]
                tunnel: w290 -> [w296]
                frame #0 {
                  n210 = call-dynamic "Write NewCommand.vi"("Command.lvclass"=w293, "System in"=w294) -> ("System out"=w295:refnum<class "Catapult.lvclass">)  [unwired: 8 in, 1 out]
                  n211 = global write "Robot Global Data.vi" "Catapult"(w295) -> ()
                }
                frame #1 {
                  n212 = call <vilib>:"Release Semaphore.vi"("error in (no error)"=w296, "semaphore"=w297) -> ()  [unwired: 4 in, 2 out]
                }
              }
            }
            frame True {
            }
          }
        }
        frame #5 {
          # "Execute Fire Catapult"
        }
      }
    }
  }
